vi "quaternion_to_axis_angle.vi"(11 "Quaternion":dbl[](array[numeric])) -> (0 "Rotation vector":dbl[](array[numeric]), 2 "Angle theta":dbl format="%.5f", 3 "Axis x":dbl[](array[numeric]))   [LabVIEW 2012]
uses:
  norm_vec.vi
panel:
  # "Given a unit quaternion, return the  axis vector and rotation angle for this 3D rotation.  The Axis is singular for small rotations, in which case we return [1, 0, 0].\n\nWe also return the rotation vector, where the angle is encoded in the magnitude."
  # "w"
  # "x1"
  # "x2"
  # "x3"
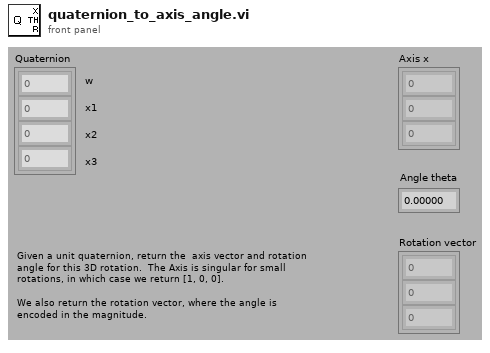
[diagram p1: front panel]
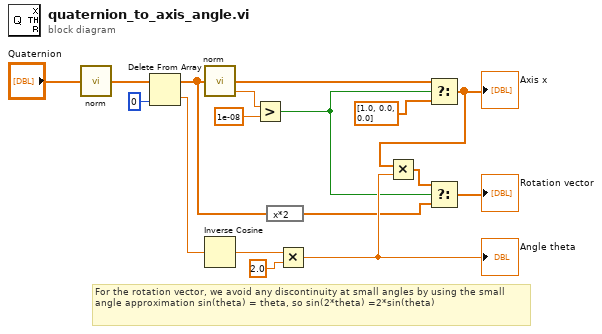
[diagram p0: block diagram]
diagram:
  # "For the rotation vector, we avoid any discontinuity at small angles by using the small angle approximation sin(theta) = theta, so sin(2*theta) =2*sin(theta)"
  n1 = call-poly "norm.vi"("vector"="Quaternion") -> ("normalized vector"=w11:dbl[])  [unwired: 3 in, 1 out]
  n2 = Delete From Array(array=w11, index=0) -> (deleted portion=w16:dbl, array with subset deleted=w5:dbl[])  [unwired: 1 in]
  n3 = call-poly "norm.vi"("vector"=w5) -> ("magnitude"=w15:dbl, "normalized vector"=w14:dbl[])  [unwired: 3 in]
  n4 = Inverse Cosine(1:w16) -> (0:w10:dbl)
  n5 = Greater?(x=w15, y=1e-08) -> (0:w3:bool)
  n6 = expression code="x*2"(w5) -> (w4:dbl[])
  n7 = Multiply(x=w10, y=2.0) -> (x*y=w9:dbl)
  "Angle theta" <- w9
  n8 = Select(t=w14, s=w3, f=dbl[] [1.0, 0.0, 0.0]) -> (s? t:f=w2:dbl[])
  "Axis x" <- w2
  n9 = Multiply(x=w2, y=w9) -> (x*y=w6:dbl[])
  n10 = Select(t=w6, s=w3, f=w4) -> (s? t:f=→"Rotation vector":dbl[])
